vi "Display Code String Core.vi"(0 "Code String LV in":refnum<class "Code String LV.lvclass">, 11 "error in (no error)":errorcluster) -> (4 "Code String LV out":refnum<class "Code String LV.lvclass">, 15 "error out":errorcluster)   [LabVIEW 2016, in "Code String LV.lvclass"]
doc: "Displays the Code String.\n--------------------\nCopyright (c) 2019 Analog Devices, Inc. All rights reserved.\n\nRedistribution and use in source and binary forms, with or without modification,\nare permitted provided that the following conditions are met:\n - Redistributions of source code must retain the above copyright notice, this\n list of conditions and the following disclaimer.\n - Redistributions in binary form must reproduce the above copyright notice,\n this list of conditions and the following disclaimer in the documentation\n and/or other materials provided with the distribution.\n - Modified versions of the software must be conspicuously marked as such.\n - This software is licensed solely and exclusively for use with\n processors/products manufactured by or for Analog Devices, Inc.\n - This software may not be combined or merged with other code in any manner\n that would cause the software to become subject to terms and conditions\n which differ from those listed here.\n - Neither the name of Analog Devices, Inc. nor the names of its contributors\n may be used to endorse or promote products derived from this software\n without specific prior written permission.\n - The use of this software may or may not infringe the patent rights of one or\n more patent holders. This license does not release you from the requirement\n that you obtain separate licenses from these patent holders to use this\n software.\n\nTHIS SOFTWARE IS PROVIDED BY ANALOG DEVICES, INC. AND CONTRIBUTORS \"AS IS\" AND\nANY EXPRESS OR IMPLIED WARRANTIES, INCLUDING, BUT NOT LIMITED TO,\nNON-INFRINGEMENT, TITLE, MERCHANTABILITY AND FITNESS FOR A PARTICULAR PURPOSE\nARE DISCLAIMED. IN NO EVENT SHALL ANALOG DEVICES, INC. OR CONTRIBUTORS BE LIABLE\nFOR ANY DIRECT, INDIRECT, INCIDENTAL, SPECIAL, EXEMPLARY, PUNITIVE OR\nCONSEQUENTIAL DAMAGES (INCLUDING, BUT NOT LIMITED TO, DAMAGES ARISING OUT OF\nCLAIMS OF INTELLECTUAL PROPERTY RIGHTS INFRINGEMENT; PROCUREMENT OF SUBSTITUTE\nGOODS OR SERVICES; LOSS OF USE, DATA, OR PROFITS; OR BUSINESS INTERRUPTION)\nHOWEVER CAUSED AND ON ANY THEORY OF LIABILITY, WHETHER IN CONTRACT, STRICT\nLIABILITY, OR TORT (INCLUDING NEGLIGENCE OR OTHERWISE) ARISING IN ANY WAY OUT OF\nTHE USE OF THIS SOFTWARE, EVEN IF ADVISED OF THE POSSIBILITY OF SUCH DAMAGE.\n\n2019-01-10-7CBSD SLA"
uses:
  Code String LV.lvclass
  C:/Git/ipn_lv_dev/code-string/source/library/Code String/Code String/Code String.lvclass
  Code String LV.lvclass/Code String LV.ctl
  Code String/Properties/Read VI.vi
panel:
  # "Copyright (c) 2019 Analog Devices, Inc.  All rights reserved.\n\nRedistribution and use in source and binary forms, with or without modification,\nare permitted provided that the following conditions are met:\n  - Redistributions of source code must retain the above copyright notice, this\n    list of conditions and the following disclaimer.\n  - Redistributions in binary form must reproduce the above copyright notice,\n    this list of conditions and the following disclaimer in the documentation\n    and/or other materials provided with the distribution.\n  - Modified versions of the software must be conspicuously marked as such.\n  - This software is licensed solely and exclusively for use with\n    processors/products manufactured by or for Analog Devices, Inc.\n  - This software may not be combined or merged with other code in any manner\n    that would cause the software to become subject to terms and conditions\n    which differ from those listed here.\n  - Neither the name of Analog Devices, Inc. nor the names of its contributors\n    may be used to endorse or promote products derived from this software\n    without specific prior written permission.\n  - The use of this software may or may not infringe the patent rights of one or\n    more patent holders.  This license does not release you from the requirement\n    that you obtain separate licenses from these patent holders to use this\n    software.\n\nTHIS SOFTWARE IS PROVIDED BY ANALOG DEVICES, INC. AND CONTRIBUTORS \"AS IS\" AND\nANY EXPRESS OR IMPLIED WARRANTIES, INCLUDING, BUT NOT LIMITED TO,\nNON-INFRINGEMENT, TITLE, MERCHANTABILITY AND FITNESS FOR A PARTICULAR PURPOSE\nARE DISCLAIMED. IN NO EVENT SHALL ANALOG DEVICES, INC. OR CONTRIBUTORS BE LIABLE\nFOR ANY DIRECT, INDIRECT, INCIDENTAL, SPECIAL, EXEMPLARY, PUNITIVE OR\nCONSEQUENTIAL DAMAGES (INCLUDING, BUT NOT LIMITED TO, DAMAGES ARISING OUT OF\nCLAIMS OF INTELLECTUAL PROPERTY RIGHTS INFRINGEMENT; PROCUREMENT OF SUBSTITUTE\nGOODS OR SERVICES; LOSS OF USE, DATA, OR PROFITS; OR BUSINESS INTERRUPTION)\nHOWEVER CAUSED AND ON ANY THEORY OF LIABILITY, WHETHER IN CONTRACT, STRICT\nLIABILITY, OR TORT (INCLUDING NEGLIGENCE OR OTHERWISE) ARISING IN ANY WAY OUT OF\nTHE USE OF THIS SOFTWARE, EVEN IF ADVISED OF THE POSSIBILITY OF SUCH DAMAGE.\n\n2019-01-10-7CBSD SLA"
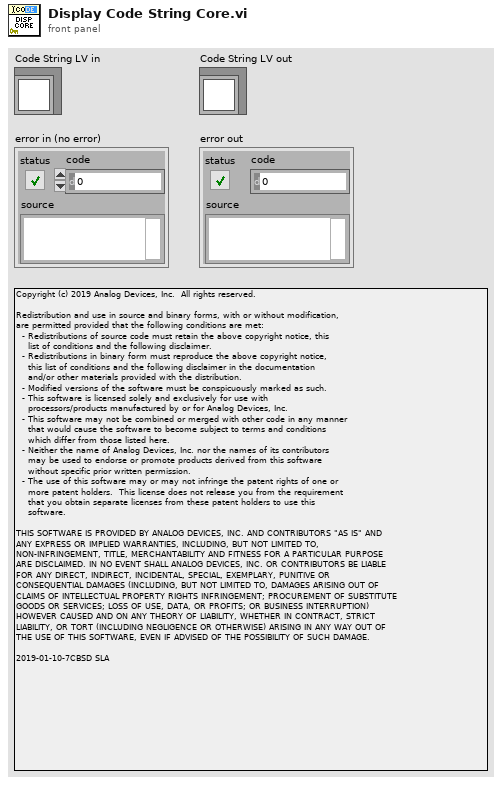
[diagram p1: front panel]
types:
  T1 = enum32{"Invalid", "Standard", "Closed", "Hidden", "Minimized", "Maximized"}
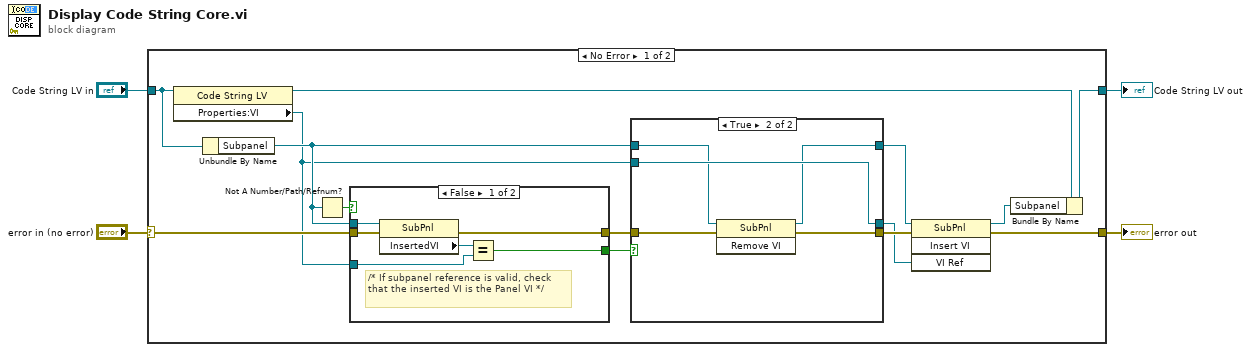
[diagram p0: block diagram]
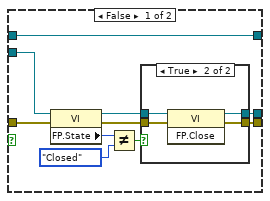
[diagram p2: hidden frame]
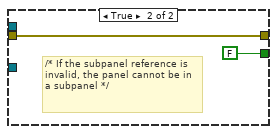
[diagram p4: hidden frame]
diagram:
  n1 = case shown="No Error" "error in (no error)" {
    selector: "error in (no error)" -> [w14 w48]
    tunnel: [w18 w48] -> w1
    tunnel: "Code String LV in" -> [w8 w49]
    tunnel: [w10 w49] -> w4
    frame No Error {
      n2 = property class="Code String LV"(reference=w8) -> (reference out=w6:refnum<class "Code String LV.lvclass">, "Properties:VI"=w5:refnum<vi>)  [unwired: 1 in, 1 out]
      n3 = Unbundle By Name(w8) -> ("Subpanel"=w11:refnum<vi>)
      n4 = Not A Number/Path/Refnum?(number/path/refnum=w11) -> (NaN/Path/Refnum?=w15:bool)
      n5 = case shown="False" w15 {
        tunnel: w11 -> [w45 _]
        tunnel: w5 -> [w44 _]
        tunnel: [w43 FALSE] -> w13
        tunnel: w14 -> [w42 w47]
        tunnel: [w41 w47] -> w12
        frame False {
          # "/* If subpanel reference is valid, check that the inserted VI is the Panel VI */"
          n6 = property class="SubPnl"(reference=w45, error in=w42) -> (error out=w41:errorcluster, "InsertedVI"=w40:refnum<vi>)  [unwired: 1 out]
          n7 = Equal?(x=w40, y=w44) -> (x = y?=w43:bool)
        }
        frame True {
          # "/* If the subpanel reference is invalid, the panel cannot be in a subpanel */"
        }
      }
      n8 = case shown="True" w13 {
        tunnel: [w28 w37] -> w17
        tunnel: [w27 w38] -> w16
        tunnel: w12 -> [w21 w39]
        tunnel: w5 -> [w20 w38]
        tunnel: w11 -> [w19 w36]
        tunnel: [w19 w35] -> w7
        frame False {
          n9 = property class="VI"(reference=w20, error in=w21) -> (reference out=w26:refnum<vi>, error out=w22:errorcluster, "FP.State"=w23:T1)
          n10 = Not Equal?(x=w23, y=T1."Closed" ("Front Panel Window:State")) -> (x != y?=w25:bool)
          n11 = case shown="True" w25 {
            tunnel: w22 -> [w30 w34]
            tunnel: [w30 w33] -> w28
            tunnel: w26 -> [w29 w32]
            tunnel: [w29 w31] -> w27
            frame False {
            }
            frame True {
              n12 = invoke class="VI" method="FP.Close"(reference=w32, error in=w34) -> (reference out=w31:refnum<vi>, error out=w33:errorcluster)  [unwired: 1 in, 1 out]
            }
          }
        }
        frame True {
          n13 = invoke class="SubPnl" method="Remove VI"(reference=w36, error in=w39) -> (reference out=w35:refnum<vi>, error out=w37:errorcluster)  [unwired: 1 in, 1 out]
        }
      }
      n14 = invoke class="SubPnl" method="Insert VI"(reference=w7, error in=w17, "VI Ref"=w16) -> (reference out=w9:refnum<vi>, error out=w18:errorcluster)  [unwired: 1 in, 2 out]
      n15 = Bundle By Name(cluster=w6, "Subpanel"=w9) -> (w10:refnum<class "Code String LV.lvclass">)
    }
    frame Error {
    }
  }
  "Code String LV out" <- w4
  "error out" <- w1
